vi "Big_LED_control.vi"() -> ()   [LabVIEW 2018]
uses:
  C:/Users/user/Desktop/LabVIEW/LED_CONTROL_big/LED_CONTROL_big_LED/AT lib/AmateurStepperMotor.dll
  AT lib/AmateurStepperMotor.dll
  <instrlib>/niDMM/nidmm.llb/niDMM Function.ctl
  <instrlib>/niDMM/nidmm.llb/niDMM Resolution in Digits.ctl
  <instrlib>/niDCPower/nidcpower.llb/niDCPower Measurement Type.ctl
  <vilib>/Instr/_visa.llb/VISA Configure Serial Port (Instr).vi
  <instrlib>/niDMM/nidmm.llb/niDMM Configure Measurement Digits.vi
panel:
  in  "Tab Control":T1(tab)
  in  "POWER":bool
  in  "Стоп":bool
  in  "Resource Name":refnum<k15>="PXI1Slot2" caption="Источник питания"
  in  "Амперметр":refnum<k15>="PXI1Slot5" caption="NI DMM 1"
  in  "V_MB, V":dbl=5.0 caption="voltage level" format="%_6p"
  in  "curlim_V_MB, A":dbl=0.3 caption="current limit" format="%_6p"
  in  "curlim_V_RESERVE, A":dbl=0.1 caption="current limit" min=0.01 format="%_6p"
  out "currentmes_V_MB, A":dbl caption="measurement" format="%_6g"
  out "currentmes_V_RESERVE, A":dbl caption="measurement" format="%_6g"
  in  "V_RESERVE, V":dbl caption="voltage level" format="%_6p"
  out "chart_2":dbl(graph)=8.556104343922883e-07
  out "chart_0":dbl(graph)=5.42616690347781e-05 caption="Waveform Chart 5"
  in  "curlim_V_LED, A":dbl=0.01 caption="current limit" min=0.01 format="%_6p"
  in  "V_LED, V":dbl=2.000000000000001 caption="voltage level" format="%_6p"
  out "chart_1":dbl(graph)=2.456762028615791e-06 caption="Waveform Chart 5"
  out "currentmes_V_LED, A":dbl caption="measurement" format="%_6g"
  in  "NI DMM 1 Current Range 3":string(combo)="1" caption="Range"
  in  "NI DMM 1 units 3":string(combo)="1000" caption="Units"
  out "Current Char":dbl(graph)=0.013612861948786303
  out "Current":dbl format="%_6g"
  in  "Arduino":refnum<visa-resource-name>="COM14"
  in  "Сегменты":bool[](array[boolean])=[FALSE, FALSE, FALSE, FALSE, FALSE, FALSE, FALSE, FALSE, FALSE, FALSE]
  in  "Вольтметр":refnum<k15>="PXI1Slot5" caption="NI DMM 1"
  in  "NI DMM 1 Voltage Range 4":string(combo)="-1" caption="Range"
  out "Voltage Char":dbl(graph)=0.013612861948786303
  in  "NI DMM 1 units 4":string(combo)="1" caption="Units"
  out "Voltage":dbl format="%_6g"
  out "Тип индикатора":string
  out "Образец №":string="0"
  in  "Ophir 1 Info":u16(ring)=1 caption="Info" items=["Device : JUNO; s/n:903793", "Head : PD300R-3W   ; s/n:779628"]
  out "Ophir 1 Initialization":bool caption="Initialization"
  out "Position":dbl
  out "Готово":bool
  in  "Стоп GoTo":bool
  in  "Погнали!":bool
  in  "Speed":dbl=1000.0
  in  "StepDivisor":i32(ring)=8 items=["D1"=1, "D2"=2, "D4"=4, "D8"=8, "D16"=16, "D32"=32]
  in  "StepMultiplicationFactor":dbl=1.0
  in  "Ophir 1 Wait":u32=100 caption="Wait"
  in  "Ophir 1 Clear":bool caption="Clear"
  out "Ophir 1 MAX":dbl caption="MAX" format="%#_5g"
  out "Ophir 1 Optical Power":dbl caption="Power" format="%#_4g"
  out "Ophir 1 Over Range":bool caption="Over Range"
  in  "Ophir 1 units":string(combo)="1000" caption="Units"
  in  "HoldOn":bool
  in  "AccelerationTime, s":dbl
  in  "DecelerationTime, s":dbl
  out "Ophir 1 Char":dbl(graph)=6.67426339573744e-05
  in  "Go To":dbl
  in  "wave_lenght":string
  in  "Port Name":string="COM1"
  in  "SEL path":path=path "D:/NI LabVIEW/MultiOpto/MultiOpto_1.2/Logs/SEL" caption="SEL Path"
  out "Разряд":dbl
  out "+/-":bool
  out "Power off":bool
  in  "Ophir 1 error in (no error)":errorcluster caption="error in (no error)"
  out "Ophir 1 error out":errorcluster caption="error out"
  in  "Ophir 1 Select Communication Protocol":u16(ring) caption="Select Communication Protocol" items=["USB", "RS232", "GPIB"]
  in  "Ophir 1 Port Number (default 2)":i16=1 caption="Port Number (default 2)" min=0 max=20
  in  "Ophir 1 GPIB Address (10)":string="10" caption="GPIB Address (10)"
  out "Ophir 1 Real Optical Power":dbl format="%.6e"
  in  "Ophir 1 Baud Rate (3:9600)":i16(ring)=3 caption="Baud Rate (3:9600)" items=["300", "1200", "4800", "9600", "19200", "38400"]
  out "Ophir 1 dup Visa Session":refnum<visa-resource-name>="USB0::0x0BD3::0x0777::NI-VISA-10003::RAW" caption="dup Visa Session"
  in  "Ophir 1 usb channel":i16 caption="usb channel"
  in  "Command":string="led_on"
  in  "Записать":bool
  out "SEL output file refnum":refnum<file>
  out "Device Response":string="*\n"
  # "V_MB 5 В\nогрничение 300 м\n\nV_LED 2,1 В\nограничение 200 м"
  # "единицы мА\nrange 1 А"
  # "единицы В\nrange AUTO"
  # "24.063\n\n     I          U\n20 мА  1.3 В\n20 мА  1.4 В\n 7 мА   1.15 В"
  # "24.064\n\n     I          U\n10 мА  2 В\n10 мА  2.15 В\n 7 мА   1.9 В"
  # "Введи ->"
  # "Р1:  +25°C\nР2:  - 60°C\nР3:  +85°C"
  # "j"
  # "c"
  # "d"
  # "e"
  # "g"
  # "h"
  # "a"
  # "b"
  # "f"
  # "k"
  # "L"
  # "m"
  # "n"
  # "p"
  # "dp"
  # "all"
  # "необходимо выдерживать 1 с между нажатиями кнопок"
  # "Шаговик"
  # "Офир"
  # "\"опрашивать кнопки не чаще, чем раз в секунду. сейчас кликать можно чаще, они загорятся, но ничего не произойдет\""
  # "Офир"
  # "автоматизировать подбор напряжения по известному максимальному напряжению и току. ОС по току сегмента"
  # "регклировка суммарного тока через индикатор"
  # "регулировать ток в зависимости от температуры.\nс ростом температуры растет ток.\nпид-регулятор??"
  # "1. каждый сегмент включаем по отдельности, резистором постраиваем ток до 10 мА\n2. напряжение V_LED при этом не меняется\n3. в такоом положении промеряем сегменты по отдельности\n4. для промера всего индикатора сразу подстраиваем напряжение при неизменном положении резисторов\n5. ток всех индикаторов = ток одного сегмента (10 мА) * число сегментов (15)\n6. добиваемся этого увеличением V_LED"
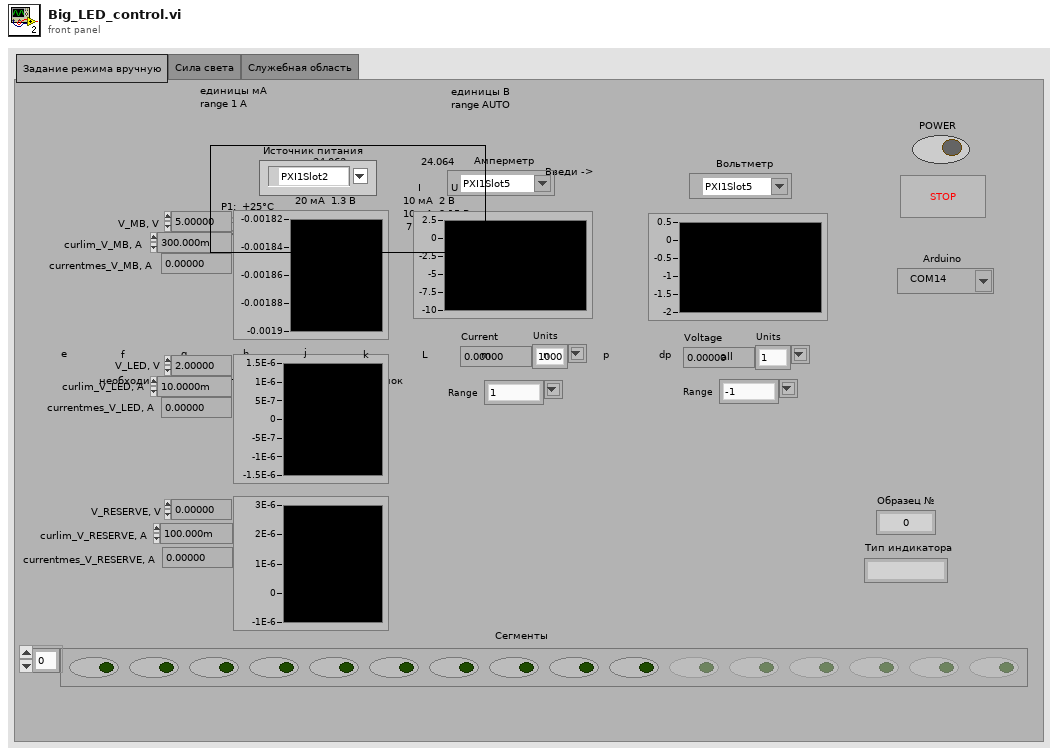
[diagram p1: front panel]
types:
  T1 = enum32{"Задание режима вручную", "Сила света", "Служебная область"}
  T2 = enum16{"open", "replace", "create", "open or create", "replace or create", "replace or create with confirmation"}
  T3 = typedef "niDCPower Measurement Type.ctl" = i32
  T4 = typedef "niDMM Function.ctl" = enum16{"DC Volts", "AC Volts", "DC Current", "AC Current", "2-wire Resistance", "4-wire Resistance", "Diode", "Frequency", "Period", "AC Volts DC Coupled", "Capacitance", "Inductance", "Temperature"}
  T5 = typedef "niDMM Resolution in Digits.ctl" = dbl
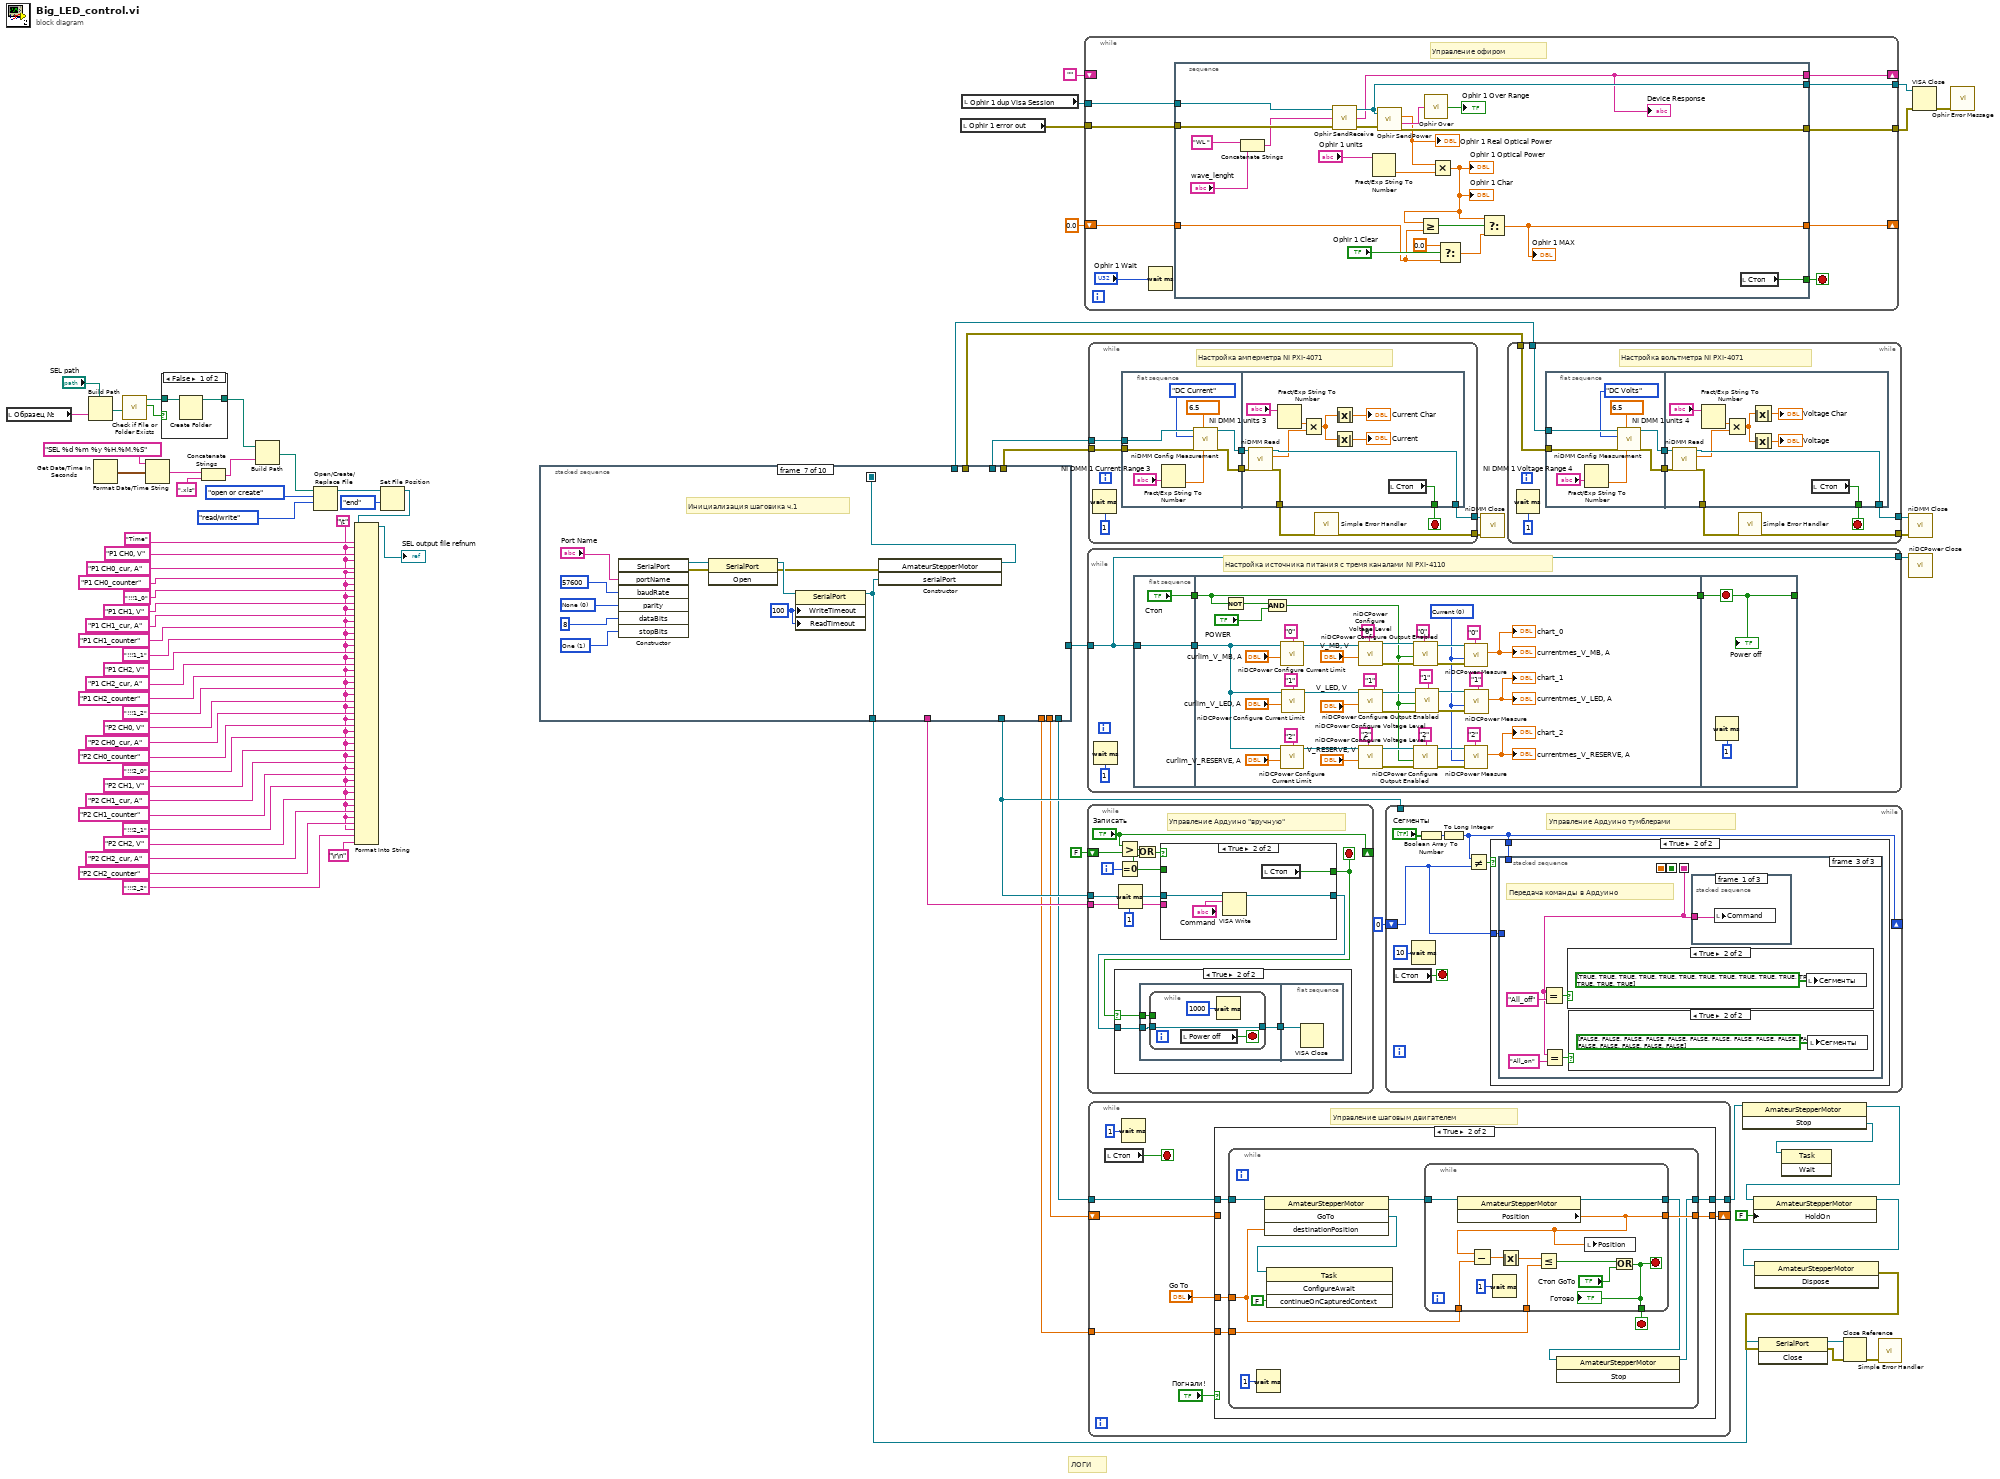
[diagram p0: block diagram]
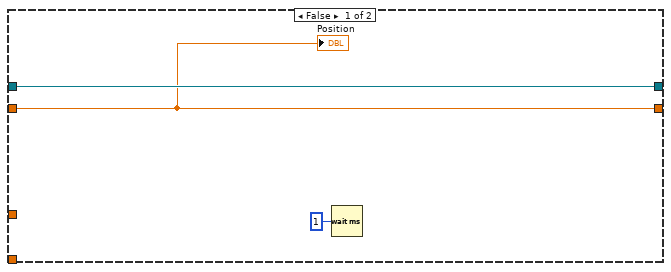
[diagram p3: hidden frame]
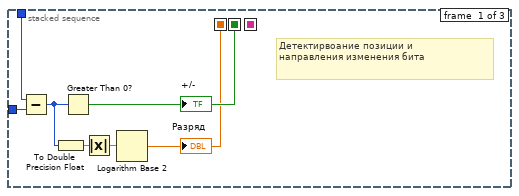
[diagram p5: hidden frame]
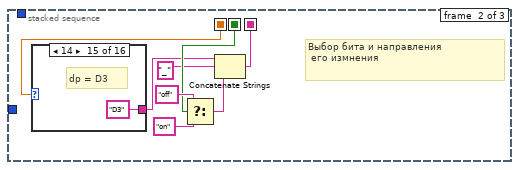
[diagram p6: hidden frame]
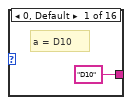
[diagram p7: hidden frame]
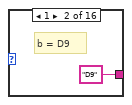
[diagram p8: hidden frame]
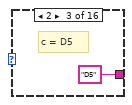
[diagram p9: hidden frame]
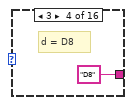
[diagram p10: hidden frame]
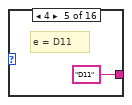
[diagram p11: hidden frame]
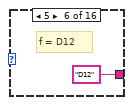
[diagram p12: hidden frame]
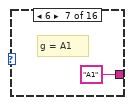
[diagram p13: hidden frame]
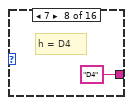
[diagram p14: hidden frame]
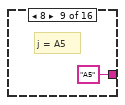
[diagram p15: hidden frame]
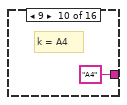
[diagram p16: hidden frame]
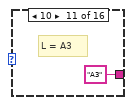
[diagram p17: hidden frame]
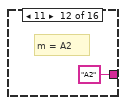
[diagram p18: hidden frame]
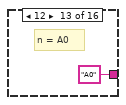
[diagram p19: hidden frame]
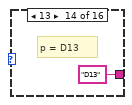
[diagram p20: hidden frame]
diagram:
  w4 = "\t"
  # "ЛОГИ"
  n1 = local read "Образец №"() -> (w31:string)
  n2 = Build Path(base path="SEL path", name or relative path=w31) -> (appended path=w46:path)
  n3 = Get Date/Time In Seconds() -> (seconds since 1Jan1904=w42:timestamp)
  n4 = call <vilib>:"Check if File or Folder Exists.vi"("path"=w46) -> ("file or folder exists?"=w45:bool, "dup path"=w44:path)  [unwired: 8 in, 1 out]
  n5 = Format Date/Time String(time format string (%c)="SEL %d %m %y %H.%M.%S", seconds (now)=w42) -> (date/time string=w41:string)  [unwired: 1 in]
  n6 = case shown="False" w45 {
    tunnel: w44 -> [w81 w82]
    tunnel: [w80 w82] -> w43
    frame False {
      n7 = Create Folder(path (use dialog)=w81) -> (created path=w80:path)  [unwired: 2 in, 2 out]
    }
    frame True {
    }
  }
  n8 = Concatenate Strings(w41, ".xls" ("string")) -> (w38:string)
  n9 = Build Path(base path=w43, name or relative path=w38) -> (appended path=w35:path)
  n10 = Open/Create/Replace File(file path (use dialog)=w35, operation (0:open)=T2."open or create", access (0:read/write)=enum16{"read/write", "read-only", "write-only"}."read/write") -> (refnum out=w34:refnum<file>)  [unwired: 3 in, 2 out]
  n11 = Set File Position(refnum=w34, from (0:start)=enum16{"start", "end", "current"}."end") -> (refnum out=w15:refnum<file>)  [unwired: 2 in, 1 out]
  n12 = Format Into String(initial string=w15, "Time" ("string"), w4, "P1 CH0, V" ("string"), w4, "P1 CH0_cur, A" ("string"), w4, "P1 CH0_counter" ("string"), w4, "!!!1_0" ("input 7"), w4, "P1 CH1, V" ("string"), w4, "P1 CH1_cur, A" ("string"), w4, "P1 CH1_counter" ("string"), w4, "!!!1_1" ("input 7"), w4, "P1 CH2, V" ("string"), w4, "P1 CH2_cur, A" ("string"), w4, "P1 CH2_counter" ("string"), w4, "!!!1_2" ("input 7"), w4, "P2 CH0, V" ("string"), w4, "P2 CH0_cur, A" ("string"), w4, "P2 CH0_counter" ("string"), w4, "!!!2_0" ("input 7"), w4, "P2 CH1, V" ("string"), w4, "P2 CH1_cur, A" ("string"), w4, "P2 CH1_counter" ("string"), w4, "!!!2_1" ("input 7"), w4, "P2 CH2, V" ("string"), w4, "P2 CH2_cur, A" ("string"), w4, "P2 CH2_counter" ("string"), w4, "!!!2_2" ("input 7"), "\r\n") -> (resulting string=→"SEL output file refnum":refnum<file>)  [unwired: 2 in, 1 out]
  n13 = stacked-sequence {
    seq-local: [_ _ _ _ _ _ w122 _ _ _] -> [_ _ _ _ _ _ _ w134 _ _]
    tunnel: [_ _ _ w93 _ _ _ _ _ _] -> w67
    tunnel: [_ w89 _ _ _ _ _ _ _ _] -> w79
    tunnel: [_ w88 _ _ _ _ _ _ _ _] -> w78
    tunnel: [_ _ _ _ w99 _ _ _ _ _] -> w75
    tunnel: [_ _ _ _ _ _ _ _ _ w144] -> w74
    tunnel: [_ _ w92 _ _ _ _ _ _ _] -> w73
    tunnel: [_ _ w91 _ _ _ _ _ _ _] -> w72
    tunnel: [_ _ _ _ _ _ _ w137 _ _] -> w66
    tunnel: [_ _ _ _ _ _ _ w135 _ _] -> w64
    tunnel: [_ _ _ _ _ _ _ w136 _ _] -> w65
    tunnel: [_ _ _ _ _ _ w123 _ _ _] -> w48
    frame #0 {
      w83 = 0.0 ("currentmes_2")
      w84 = FALSE ("Стоп")
      # "Обнуление переменных"
      n14 = local write "POWER"(w84) -> ()
      n15 = local write "Стоп"(w84) -> ()
      n16 = local write "+/-"(w84) -> ()
      n17 = local write "Погнали!"(w84) -> ()
      n18 = local write "Готово"(w84) -> ()
      n19 = local write "Стоп GoTo"(w84) -> ()
      n20 = local write "currentmes_V_MB, A"(w83) -> ()
      n21 = local write "currentmes_V_LED, A"(w83) -> ()
      n22 = local write "currentmes_V_RESERVE, A"(w83) -> ()
      n23 = local write "Current"(w83) -> ()
      n24 = local write "Разряд"(w83) -> ()
      n25 = local write "Go To"(w83) -> ()
      n26 = local write "Сегменты"(bool[] [FALSE, FALSE, FALSE, FALSE, FALSE, FALSE, FALSE, FALSE, FALSE, FALSE, FALSE, FALSE, FALSE, FALSE, FALSE, FALSE, FALSE, FALSE] ("Сегменты")) -> ()
      n27 = local write "Command"("zero" ("Command 2")) -> ()
    }
    frame #1 {
      # "Инициализация амперметра"
      n28 = call <instrlib>:"niDMM Initialize.vi"("Instrument Descriptor"="Амперметр") -> ("error out"=w89:errorcluster, "instrument handle out"=w88:refnum<k15>)  [unwired: 9 in]
    }
    frame #2 {
      # "Инициализация вольтметра"
      n29 = call <instrlib>:"niDMM Initialize.vi"("Instrument Descriptor"="Вольтметр") -> ("error out"=w91:errorcluster, "instrument handle out"=w92:refnum<k15>)  [unwired: 9 in]
    }
    frame #3 {
      # "Инициализация источника питания"
      n30 = call <instrlib>:"niDCPower Initialize.vi"("resource name"="Resource Name") -> ("error out"=w95:errorcluster, "instrument handle out"=w96:refnum<k15>)  [unwired: 3 in, 6 out]
      n31 = call <instrlib>:"niDCPower Configure Voltage Level.vi"("error in (no error)"=w95, "voltage level"=0.0, "channel name"="0,1,2", "instrument handle"=w96) -> ("instrument handle out"=w93:refnum<k15>)  [unwired: 6 in, 1 out]
    }
    frame #4 {
      # "Инициализация Ардуино"
      n32 = call-poly "VISA Configure Serial Port"("VISA resource name"="Arduino", "baud rate (9600)"=u32 9600) -> ("VISA resource name out"=w99:refnum<visa-resource-name>)  [unwired: 12 in, 1 out]
    }
    frame #5 {
      # "Инициализация офира"
      n33 = call "Ophir InitCom.vi"("GPIB Address (default 10)"="Ophir 1 GPIB Address (10)", "Communication (default USB 0)"="Ophir 1 Select Communication Protocol", "USB Channel number (default 0)"="Ophir 1 usb channel", "Port Number (default 2)"="Ophir 1 Port Number (default 2)", "error in (no error)"="Ophir 1 error in (no error)", "Baud Rate (3:9600)"="Ophir 1 Baud Rate (3:9600)") -> ("dup Visa Session"=w108:refnum<visa-resource-name>, "error out"=w107:errorcluster)  [unwired: 1 out]
      n34 = call "Ophir InstrInfo.vi"("Visa Session"=w108, "error in (no error)"=w107) -> ("dup Visa Session"=w120:refnum<visa-resource-name>, "Instrument Info"=w102:string, "error out"=w118:errorcluster)
      n35 = call "Ophir HeadInfo.vi"("Visa Session"=w120, "error in (no error)"=w118) -> ("error out"=w117:errorcluster, "dup Visa Session"=w119:refnum<visa-resource-name>, "Head Info"=w116:string)  [unwired: 6 out]
      n36 = call "Ophir InfoStrings.vi"("error in (no error)"=w117, "Head Info"=w116, "Instrument Info"=w102) -> ("error out"=w115:errorcluster, "Strings Array"=w114:string[])
      n37 = property on="Ophir 1 Info" class="Ring (strict)"("Strings []"=w114) -> ()  [unwired: 2 in, 2 out]
      n38 = call "Ophir ConfigDevice.vi"("Visa Session"=w119, "Measure Choice (0:Power)"=u16 0, "error in (no error)"=w115) -> ("dup Visa Session"=→"Ophir 1 dup Visa Session":refnum<visa-resource-name>, "OK ?"=→"Ophir 1 Initialization":bool, "error out"=→"Ophir 1 error out":errorcluster)  [unwired: 1 out]
    }
    frame #6 {
      w126 = 100 ("WriteTimeout")
      w133 = 1 items=["None", "One", "Two", "OnePointFive"] ("stopBits")
      w130 = 0 items=["None", "Odd", "Even", "Mark", "Space"] ("parity")
      # "Инициализация шаговика ч.1"
      n39 = constructor class="SerialPort"("portName"="Port Name", "baudRate"=57600, "parity"=w130, "dataBits"=8, "stopBits"=w133) -> (reference out=w128:refnum<k24>, error out=w127:errorcluster)  [unwired: 3 in, 6 out]
      n40 = invoke class="SerialPort" method="Open"(reference=w128, error in=w127) -> (reference out=w125:refnum<k24>, error out=w124:errorcluster)  [unwired: 1 in, 1 out]
      n41 = property class="SerialPort"(reference=w125, "WriteTimeout"=w126, "ReadTimeout"=w126) -> (reference out=w123:refnum<k24>)  [unwired: 1 in, 1 out]
      n42 = constructor class="AmateurStepperMotor"(error in=w124, "serialPort"=w123) -> (reference out=w122:refnum<k24>)  [unwired: 2 in, 3 out]
    }
    frame #7 {
      # "Инициализация шаговика ч.2"
      n43 = property class="AmateurStepperMotor"(reference=w134, "Speed"="Speed", "StepDivisor"="StepDivisor", "StepMultiplicationFactor"="StepMultiplicationFactor", "AccelerationTime"="AccelerationTime, s", "DecelerationTime"="DecelerationTime, s", "HoldOn"="HoldOn") -> (reference out=w137:refnum<k24>, "Position"=w135:dbl, "PositioningPrecision"=w136:dbl)  [unwired: 1 in, 1 out]
    }
    frame #8 {
      # "Инициализация логов"
    }
    frame #9 {
      # "Begin VI: ОК или ОА?"
      n44 = call "Begin.vi"() -> ("String"=w144:string)  [unwired: 8 in]
      "Тип индикатора" <- w144
      n45 = local write "Command"(w144) -> ()
    }
  }
  n46 = local read "Ophir 1 error out"() -> (w62:errorcluster)
  n47 = local read "Ophir 1 dup Visa Session"() -> (w63:refnum<visa-resource-name>)
  n48 = while {
    tunnel: [w153] -> w58
    tunnel: [w147] -> w59
    tunnel: w63 -> [w151]
    tunnel: w62 -> [w150]
    shift-right: [w148] -> _
    shift-left: 0.0 ("t") -> [w149]
    shift-right: [w145] -> _
    shift-left: "" -> [_]
    stop <- w152 stop-if-true
    # "Управление офиром"
    n49 = Wait (ms)(milliseconds to wait="Ophir 1 Wait") -> ()  [unwired: 1 out]
    n50 = stacked-sequence {
      tunnel: [w175] -> w153
      tunnel: [w162] -> w152
      tunnel: w151 -> [w159]
      tunnel: w150 -> [w158]
      tunnel: w149 -> [w166]
      tunnel: [w164] -> w148
      tunnel: [w160] -> w147
      tunnel: [w154] -> w145
      frame #0 {
        n51 = Concatenate Strings("WL " ("string"), "wave_lenght") -> (w155:string)
        n52 = call "Ophir SendReceive.vi"("error in (no error)"=w158, "Command"=w155, "Visa Session"=w159) -> ("error out"=w161:errorcluster, "Frame Output"=w154:string, "dup Visa Session"=w160:refnum<visa-resource-name>)
        "Device Response" <- w154
        n53 = Fract/Exp String To Number(string="Ophir 1 units") -> (number=w165:dbl)  [unwired: 3 in, 1 out]
        n54 = call "Ophir SendPower.vi"("Visa Session"=w160, "error in (no error)"=w161) -> ("Value Number"=w163:dbl, "Value String"=w173:string, "error out"=w175:errorcluster)  [unwired: 1 out]
        "Ophir 1 Real Optical Power" <- w163
        n55 = call "Ophir Over.vi"("Value String"=w173) -> ("Overrange"=→"Ophir 1 Over Range":bool)
        n56 = Multiply(x=w163, y=w165) -> (x*y=w170:dbl)
        "Ophir 1 Char" <- w170
        "Ophir 1 Optical Power" <- w170
        n57 = Greater Or Equal?(x=w170, y=w166) -> (x >= y?=w171:bool)
        n58 = Select(t=0.0, s="Ophir 1 Clear", f=w166) -> (s? t:f=w169:dbl)
        n59 = Select(t=w170, s=w171, f=w169) -> (s? t:f=w164:dbl)
        "Ophir 1 MAX" <- w164
        n60 = local read "Стоп"() -> (w162:bool)
      }
    }
  }
  n61 = while {
    tunnel: w67 -> [w177]
    tunnel: [w177] -> w76
    stop <- w178 stop-if-true
    # "Настройка источника питания с тремя каналами NI PXI-4110"
    n62 = Wait (ms)(milliseconds to wait=u32 1) -> ()  [unwired: 1 out]
    n63 = flat-sequence {
      tunnel: w177 -> [w183]
      tunnel: [w183] -> w180
      tunnel: ["Стоп"] -> w179
      tunnel: w180 -> [w191]
      tunnel: w179 -> [w225]
      tunnel: [w225] -> w176
      tunnel: [w227] -> w178
      tunnel: w176 -> [w227]
      frame #0 {
      }
      frame #1 {
        w190 = T3 0 items=["Current", "Voltage"] ("measurement type")
        n64 = Not(x=w225) -> (.not. x?=w224:bool)
        n65 = And(x=w224, y="POWER") -> (x .and. y?=w186:bool)
        n66 = call <instrlib>:"niDCPower Configure Current Limit.vi"("current limit"="curlim_V_MB, A", "channel name"="0", "instrument handle"=w191) -> ("instrument handle out"=w210:refnum<k15>)  [unwired: 7 in, 1 out]
        n67 = call <instrlib>:"niDCPower Configure Current Limit.vi"("current limit"="curlim_V_RESERVE, A", "channel name"="2", "instrument handle"=w191) -> ("instrument handle out"=w209:refnum<k15>)  [unwired: 7 in, 1 out]
        n68 = call <instrlib>:"niDCPower Configure Current Limit.vi"("current limit"="curlim_V_LED, A", "channel name"="1", "instrument handle"=w191) -> ("instrument handle out"=w218:refnum<k15>)  [unwired: 7 in, 1 out]
        n69 = call <instrlib>:"niDCPower Configure Voltage Level.vi"("voltage level"="V_MB, V", "channel name"="0", "instrument handle"=w210) -> ("error out"=w215:errorcluster, "instrument handle out"=w212:refnum<k15>)  [unwired: 7 in]
        n70 = call <instrlib>:"niDCPower Configure Voltage Level.vi"("voltage level"="V_LED, V", "channel name"="1", "instrument handle"=w218) -> ("error out"=w221:errorcluster, "instrument handle out"=w219:refnum<k15>)  [unwired: 7 in]
        n71 = call <instrlib>:"niDCPower Configure Voltage Level.vi"("voltage level"="V_RESERVE, V", "channel name"="2", "instrument handle"=w209) -> ("error out"=w214:errorcluster, "instrument handle out"=w213:refnum<k15>)  [unwired: 7 in]
        n72 = call <instrlib>:"niDCPower Configure Output Enabled.vi"("error in (no error)"=w215, "output enabled"=w186, "channel name"="0", "instrument handle"=w212) -> ("error out"=w205:errorcluster, "instrument handle out"=w206:refnum<k15>)  [unwired: 6 in]
        n73 = call <instrlib>:"niDCPower Configure Output Enabled.vi"("error in (no error)"=w214, "output enabled"=w186, "channel name"="2", "instrument handle"=w213) -> ("error out"=w204:errorcluster, "instrument handle out"=w203:refnum<k15>)  [unwired: 6 in]
        n74 = call <instrlib>:"niDCPower Configure Output Enabled.vi"("error in (no error)"=w221, "output enabled"=w186, "channel name"="1", "instrument handle"=w219) -> ("error out"=w222:errorcluster, "instrument handle out"=w220:refnum<k15>)  [unwired: 6 in]
        n75 = call <instrlib>:"niDCPower Measure.vi"("error in (no error)"=w205, "measurement type"=w190, "channel name"="0", "instrument handle"=w206) -> ("measurement"=→"currentmes_V_MB, A" →"chart_0":dbl)  [unwired: 5 in, 2 out]
        n76 = call <instrlib>:"niDCPower Measure.vi"("error in (no error)"=w204, "measurement type"=w190, "channel name"="2", "instrument handle"=w203) -> ("measurement"=→"currentmes_V_RESERVE, A" →"chart_2":dbl)  [unwired: 5 in, 2 out]
        n77 = call <instrlib>:"niDCPower Measure.vi"("error in (no error)"=w222, "measurement type"=w190, "channel name"="1", "instrument handle"=w220) -> ("measurement"=→"chart_1" →"currentmes_V_LED, A":dbl)  [unwired: 5 in, 2 out]
      }
      frame #2 {
        n78 = Wait (ms)(milliseconds to wait=u32 1) -> ()  [unwired: 1 out]
        "Power off" <- w227
      }
    }
  }
  n79 = while {
    tunnel: w75 -> [w235]
    shift-right: ["Записать"] -> _
    shift-left: FALSE ("Записать") -> [w237]
    tunnel: w74 -> [w233]
    i -> [w234]
    stop <- w228 stop-if-true
    # "Управление Ардуино \"вручную\""
    n80 = Greater?(x="Записать", y=w237) -> (0:w231:bool)
    n81 = Equal To 0?(x=w234) -> (x = 0?=w230:bool)
    n82 = Wait (ms)(milliseconds to wait=u32 1) -> ()  [unwired: 1 out]
    n83 = Or(x=w231, y=w230) -> (x .or. y?=w232:bool)
    n84 = case shown="True" w232 {
      tunnel: w235 -> [w249 w254]
      tunnel: [w250 w253] -> w228
      tunnel: w233 -> [_ _]
      tunnel: w230 -> [_ _]
      tunnel: [w249 w251] -> w229
      frame False {
        n85 = local read "Стоп"() -> (w250:bool)
      }
      frame True {
        n86 = VISA Write(VISA resource name=w254, write buffer="Command") -> (VISA resource name out=w251:refnum<visa-resource-name>)  [unwired: 1 in, 2 out]
        n87 = local read "Стоп"() -> (w253:bool)
      }
    }
    n88 = case shown="True" w228 {
      selector: w228 -> [_ w239]
      tunnel: w229 -> [_ w241]
      frame False {
      }
      frame True {
        n89 = flat-sequence {
          tunnel: w241 -> [w244]
          tunnel: [w243] -> w240
          tunnel: w239 -> [w242]
          tunnel: w240 -> [w248]
          frame #0 {
            n90 = while {
              tunnel: w244 -> [w247]
              tunnel: [w247] -> w243
              tunnel: w242 -> [_]
              stop <- w245 stop-if-true
              n91 = local read "Power off"() -> (w245:bool)
              n92 = Wait (ms)(milliseconds to wait=u32 1000) -> ()  [unwired: 1 out]
            }
          }
          frame #1 {
            n93 = VISA Close(VISA resource name=w248) -> ()  [unwired: 1 in, 1 out]
          }
        }
      }
    }
  }
  n94 = while {
    tunnel: [w261] -> w68
    tunnel: w78 -> [w259]
    tunnel: w79 -> [w258]
    tunnel: [w255] -> w69
    stop <- w257 stop-if-true
    # "Настройка амперметра NI PXI-4071"
    n95 = Wait (ms)(milliseconds to wait=u32 1) -> ()  [unwired: 1 out]
    n96 = flat-sequence {
      tunnel: [w268] -> w263
      tunnel: w259 -> [w266]
      tunnel: w258 -> [w270]
      tunnel: [w267] -> w262
      tunnel: w263 -> [w279]
      tunnel: w262 -> [w282]
      tunnel: [w278] -> w257
      tunnel: [w277] -> w255
      tunnel: [w276] -> w256
      frame #0 {
        w264 = T5 6.5 items=["3 1/2"=3.5, "4 1/2"=4.5, "5 1/2"=5.5, "6 1/2"=6.5, "7 1/2"=7.5] ("Resolution in Digits")
        n97 = Fract/Exp String To Number(string="NI DMM 1 Current Range 3") -> (number=w269:dbl)  [unwired: 3 in, 1 out]
        n98 = call-poly <instrlib>:"niDMM Config Measurement.vi"("Range"=w269, "Resolution in Digits"=w264, "error in (no error)"=w270, "Function"=niDMM_Function."DC Current" ("Measurement Type"), "instrument handle"=w266) -> ("error out"=w267:errorcluster, "instrument handle out"=w268:refnum<k15>)  [unwired: 5 in]
      }
      frame #1 {
        n99 = call <instrlib>:"niDMM Read.vi"("error in (no error)"=w282, "instrument handle"=w279) -> ("error out"=w276:errorcluster, "Measurement"=w274:dbl, "instrument handle out"=w277:refnum<k15>)  [unwired: 7 in]
        n100 = Fract/Exp String To Number(string="NI DMM 1 units 3") -> (number=w280:dbl)  [unwired: 3 in, 1 out]
        n101 = Multiply(x=w280, y=w274) -> (x*y=w272:dbl)
        n102 = Absolute Value(x=w272) -> (abs(x)=→"Current Char":dbl)
        n103 = Absolute Value(x=w272) -> (abs(x)=→"Current":dbl)
        n104 = local read "Стоп"() -> (w278:bool)
      }
    }
    n105 = call <vilib>:"Simple Error Handler.vi"("error in (no error)"=w256) -> ("error out"=w261:errorcluster)  [unwired: 1 in, 7 out]
  }
  n106 = while {
    tunnel: w66 -> [w291]
    tunnel: w65 -> [w288]
    shift-right: [w287] -> _
    shift-left: w64 -> [w290]
    tunnel: [w286] -> w55
    stop <- w284 stop-if-true
    # "Управление шаговым двигателем"
    n107 = local read "Стоп"() -> (w284:bool)
    n108 = Wait (ms)(milliseconds to wait=u32 1) -> ()  [unwired: 1 out]
    n109 = case shown="True" "Погнали!" {
      tunnel: "Go To" -> [_ w299]
      tunnel: w291 -> [w293 w298]
      tunnel: [w293 w297] -> w286
      tunnel: w290 -> [w292 _]
      tunnel: [w292 w296] -> w287
      tunnel: w288 -> [_ w295]
      frame False {
        n110 = Wait (ms)(milliseconds to wait=u32 1) -> ()  [unwired: 1 out]
        "Position" <- w292
      }
      frame True {
        n111 = while {
          tunnel: w299 -> [w305]
          tunnel: w298 -> [w306]
          tunnel: [w302] -> w297
          tunnel: [w310] -> w296
          tunnel: w295 -> [w308]
          stop <- w309 stop-if-true
          n112 = Wait (ms)(milliseconds to wait=u32 1) -> ()  [unwired: 1 out]
          n113 = invoke class="AmateurStepperMotor" method="GoTo"(reference=w306, "destinationPosition"=w305) -> (reference out=w300:refnum<k24>, "GoTo"=w304:refnum<k24>)  [unwired: 2 in, 2 out]
          n114 = invoke class="Task" method="ConfigureAwait"(reference=w304, "continueOnCapturedContext"=FALSE) -> ()  [unwired: 2 in, 4 out]
          n115 = while {
            tunnel: [w313] -> w310
            tunnel: [w312] -> w301
            tunnel: [w315] -> w309
            tunnel: w305 -> [w320]
            tunnel: w308 -> [w318]
            tunnel: w300 -> [w311]
            stop <- w315 stop-if-true
            n116 = property class="AmateurStepperMotor"(reference=w311) -> (reference out=w312:refnum<k24>, "Position"=w313:dbl)  [unwired: 1 in, 1 out]
            n117 = Subtract(x=w313, y=w320) -> (x-y=w321:dbl)
            n118 = Wait (ms)(milliseconds to wait=u32 1) -> ()  [unwired: 1 out]
            n119 = Absolute Value(x=w321) -> (abs(x)=w319:dbl)
            n120 = Less Or Equal?(x=w319, y=w318) -> (x <= y?=w317:bool)
            n121 = local write "Position"(w313) -> ()
            n122 = Or(x=w317, y="Стоп GoTo") -> (x .or. y?=w315:bool)
            "Готово" <- w315
          }
          n123 = invoke class="AmateurStepperMotor" method="Stop"(reference=w301) -> (reference out=w302:refnum<k24>)  [unwired: 2 in, 2 out]
        }
      }
    }
  }
  n124 = while {
    shift-right: [w324] -> _
    shift-left: 0 -> [w325]
    tunnel: w75 -> [_]
    stop <- w328 stop-if-true
    # "Управление Ардуино тумблерами"
    n125 = local read "Стоп"() -> (w328:bool)
    n126 = Wait (ms)(milliseconds to wait=u32 10 ("millisecond timer value")) -> ()  [unwired: 1 out]
    n127 = Boolean Array To Number(Boolean array="Сегменты") -> (number=w323:u32)
    n128 = To Long Integer(number=w323) -> (32bit integer=w324:i32)
    n129 = Not Equal?(x=w324, y=w325) -> (x != y?=w326:bool)
    n130 = case shown="True" w326 {
      tunnel: w324 -> [_ w329]
      tunnel: w325 -> [_ w330]
      frame False {
      }
      frame True {
        n131 = stacked-sequence {
          seq-local: [w333 _ _] -> [_ w343 _]
          seq-local: [w331 _ _] -> [_ w338 _]
          seq-local: [_ w339 _] -> [_ _ w363]
          tunnel: w329 -> [w335 _ _]
          tunnel: w330 -> [w334 _ _]
          frame #0 {
            # "Детектирвоание позиции и\nнаправления изменения бита"
            n132 = Subtract(x=w335, y=w334) -> (x-y=w336:i32)
            n133 = To Double Precision Float(number=w336) -> (double precision float=w337:dbl)
            n134 = Greater Than 0?(x=w336) -> (x > 0?=w333:bool)
            "+/-" <- w333
            n135 = Absolute Value(x=w337) -> (abs(x)=w332:dbl)
            n136 = Logarithm Base 2(1:w332) -> (0:w331:dbl)
            "Разряд" <- w331
          }
          frame #1 {
            # "Выбор бита и направления\n его измнения"
            n137 = case shown="14" w338 {
              tunnel: ["D10" "D9" "D5" "D8" "D11" "D12" "A1" "D4" "A5" "A4" "A3" "A2" "A0" "D13" "D3" "All"] -> w341
              frame 0, Default {
                # "a = D10"
              }
              frame 1 {
                # "b = D9"
              }
              frame 2 {
                # "c = D5"
              }
              frame 3 {
                # "d = D8"
              }
              frame 4 {
                # "e = D11"
              }
              frame 5 {
                # "f = D12"
              }
              frame 6 {
                # "g = A1"
              }
              frame 7 {
                # "h = D4"
              }
              frame 8 {
                # "j = A5"
              }
              frame 9 {
                # "k = A4"
              }
              frame 10 {
                # "L = A3"
              }
              frame 11 {
                # "m = A2"
              }
              frame 12 {
                # "n = A0"
              }
              frame 13 {
                # "p = D13"
              }
              frame 14 {
                # "dp = D3"
              }
              frame 15 {
              }
            }
            n138 = Select(t="off", s=w343, f="on") -> (s? t:f=w340:string)
            n139 = Concatenate Strings(w341, "_" ("string"), w340) -> (w339:string)
          }
          frame #2 {
            # "Передача команды в Ардуино"
            n140 = Equal?(x=w363, y="All_off") -> (x = y?=w366:bool)
            n141 = Equal?(x=w363, y="All_on") -> (x = y?=w364:bool)
            n142 = case shown="True" w366 {
              frame False {
              }
              frame True {
                n143 = local write "Сегменты"(bool[] [TRUE, TRUE, TRUE, TRUE, TRUE, TRUE, TRUE, TRUE, TRUE, TRUE, TRUE, TRUE, TRUE, TRUE, TRUE, TRUE] ("Сегменты")) -> ()
              }
            }
            n144 = case shown="True" w364 {
              frame False {
              }
              frame True {
                n145 = local write "Сегменты"(bool[] [FALSE, FALSE, FALSE, FALSE, FALSE, FALSE, FALSE, FALSE, FALSE, FALSE, FALSE, FALSE, FALSE, FALSE, FALSE, FALSE] ("Сегменты")) -> ()
              }
            }
            n146 = stacked-sequence {
              tunnel: w363 -> [w369 _ _]
              frame #0 {
                n147 = local write "Command"(w369) -> ()
              }
              frame #1 {
                n148 = local write "Записать"(TRUE ("Записать")) -> ()
                n149 = Wait (ms)(milliseconds to wait=u32 1000) -> ()  [unwired: 1 out]
              }
              frame #2 {
                n150 = local write "Записать"(FALSE ("Записать")) -> ()
                n151 = Wait (ms)(milliseconds to wait=u32 1000) -> ()  [unwired: 1 out]
              }
            }
          }
        }
      }
    }
  }
  n152 = call <instrlib>:"niDMM Close.vi"("error in (no error)"=w68, "instrument handle"=w69) -> ()  [unwired: 9 in, 1 out]
  n153 = while {
    tunnel: [w380] -> w70
    tunnel: w73 -> [w378]
    tunnel: w72 -> [w377]
    tunnel: [w374] -> w71
    stop <- w376 stop-if-true
    # "Настройка вольтметра NI PXI-4071"
    n154 = Wait (ms)(milliseconds to wait=u32 1) -> ()  [unwired: 1 out]
    n155 = flat-sequence {
      tunnel: [w387] -> w382
      tunnel: w378 -> [w385]
      tunnel: w377 -> [w389]
      tunnel: [w386] -> w381
      tunnel: w382 -> [w398]
      tunnel: w381 -> [w401]
      tunnel: [w397] -> w376
      tunnel: [w396] -> w374
      tunnel: [w395] -> w375
      frame #0 {
        w383 = T5 6.5 items=["3 1/2"=3.5, "4 1/2"=4.5, "5 1/2"=5.5, "6 1/2"=6.5, "7 1/2"=7.5] ("Resolution in Digits")
        n156 = Fract/Exp String To Number(string="NI DMM 1 Voltage Range 4") -> (number=w388:dbl)  [unwired: 3 in, 1 out]
        n157 = call-poly <instrlib>:"niDMM Config Measurement.vi"("Range"=w388, "Resolution in Digits"=w383, "error in (no error)"=w389, "Function"=niDMM_Function."DC Volts" ("Measurement Type"), "instrument handle"=w385) -> ("error out"=w386:errorcluster, "instrument handle out"=w387:refnum<k15>)  [unwired: 5 in]
      }
      frame #1 {
        n158 = call <instrlib>:"niDMM Read.vi"("error in (no error)"=w401, "instrument handle"=w398) -> ("error out"=w395:errorcluster, "Measurement"=w393:dbl, "instrument handle out"=w396:refnum<k15>)  [unwired: 7 in]
        n159 = Fract/Exp String To Number(string="NI DMM 1 units 4") -> (number=w399:dbl)  [unwired: 3 in, 1 out]
        n160 = Multiply(x=w399, y=w393) -> (x*y=w391:dbl)
        n161 = Absolute Value(x=w391) -> (abs(x)=→"Voltage Char":dbl)
        n162 = Absolute Value(x=w391) -> (abs(x)=→"Voltage":dbl)
        n163 = local read "Стоп"() -> (w397:bool)
      }
    }
    n164 = call <vilib>:"Simple Error Handler.vi"("error in (no error)"=w375) -> ("error out"=w380:errorcluster)  [unwired: 1 in, 7 out]
  }
  n165 = invoke class="AmateurStepperMotor" method="Stop"(reference=w55) -> (reference out=w53:refnum<k24>, "Stop"=w54:refnum<k24>)  [unwired: 2 in, 1 out]
  n166 = property class="AmateurStepperMotor"(reference=w53, "HoldOn"=FALSE) -> (reference out=w52:refnum<k24>)  [unwired: 1 in, 1 out]
  n167 = invoke class="AmateurStepperMotor" method="Dispose"(reference=w52) -> (error out=w49:errorcluster)  [unwired: 2 in, 2 out]
  n168 = invoke class="SerialPort" method="Close"(reference=w48, error in=w49) -> (reference out=w47:refnum<k24>, error out=w50:errorcluster)  [unwired: 1 in, 1 out]
  n169 = invoke class="Task" method="Wait"(reference=w54) -> ()  [unwired: 2 in, 3 out]
  n170 = Close Reference(reference=w47, error in (no error)=w50) -> (error out=w51:errorcluster)
  n171 = call <vilib>:"Simple Error Handler.vi"("error in (no error)"=w51) -> ()  [unwired: 1 in, 8 out]
  n172 = call <instrlib>:"niDMM Close.vi"("error in (no error)"=w70, "instrument handle"=w71) -> ()  [unwired: 9 in, 1 out]
  n173 = call <instrlib>:"niDCPower Close.vi"("instrument handle"=w76) -> ()  [unwired: 10 in, 1 out]
  n174 = VISA Close(VISA resource name=w59, error in (no error)=w58) -> (error out=w60:errorcluster)
  n175 = call "Ophir Error Message.vi"("error in (no error)"=w60) -> ()  [unwired: 3 in, 4 out]
